vi "Translate Hub Coords.vi"(8 "TOF":dbl, 10 "Input Velocities":T1, 11 "Hub Coords":cluster{"X":dbl, "Y":dbl}) -> (2 "Distance to Hub (ft)":dbl, 3 "Hub Coords Out":cluster{"X":dbl, "Y":dbl})   [LabVIEW 2025]
uses:
  swerve-template/Type Definitions/Data/Robot Velocities.ctl
panel:
  out "Waveform Chart 2":cluster{"Numeric":sgl, "Numeric":sgl}(graph)
  out "Waveform Chart":dbl(graph)
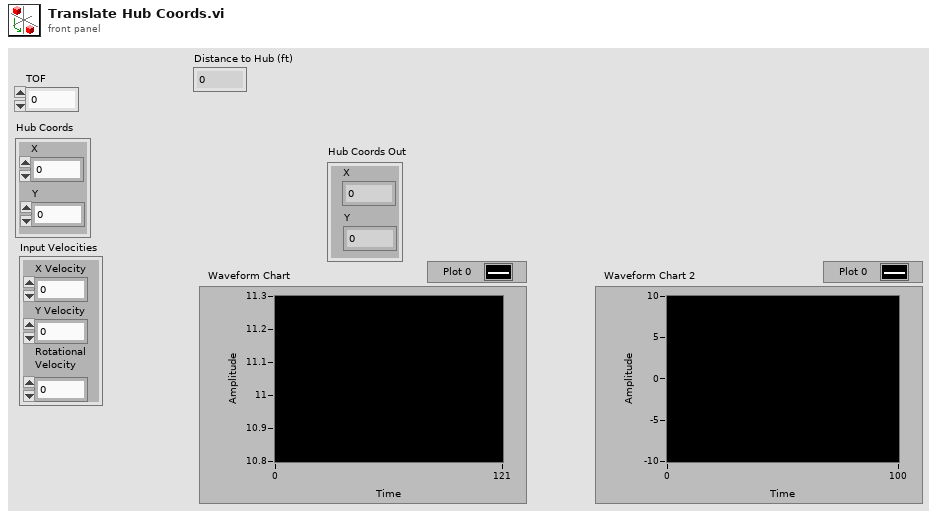
[diagram p1: front panel]
types:
  T1 = typedef "Robot Velocities.ctl" = cluster{"X Velocity":dbl, "Y Velocity":dbl, "Rotational \nVelocity":dbl}
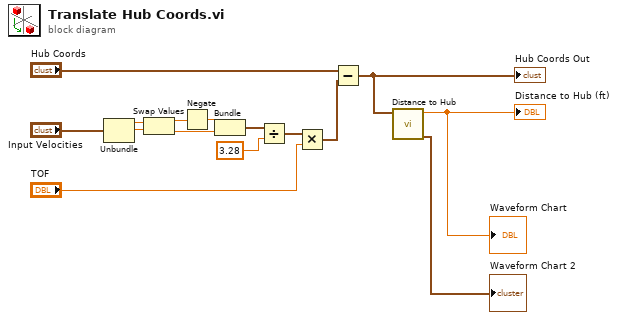
[diagram p0: block diagram]
diagram:
  n1 = Unbundle("Input Velocities") -> ("X Velocity"=w8:dbl, "Y Velocity"=w7:dbl)  [unwired: 1 out]
  n2 = Swap Values(12:w8, 14:w7) -> (1:w4:dbl, 3:w6:dbl)  [unwired: 1 in]
  n3 = Negate(x=w4) -> (-x=w3:dbl)
  n4 = Bundle(w3, w6) -> (w5:cluster{dbl, dbl})  [unwired: 1 in]
  n5 = Divide(x=w5, y=3.28) -> (x/y=w13:cluster{dbl, dbl})
  n6 = Multiply(x=w13, y="TOF") -> (x*y=w9:cluster{dbl, dbl})
  n7 = Subtract(x="Hub Coords", y=w9) -> (x-y=w10:cluster{dbl, dbl})
  "Hub Coords Out" <- w10
  n8 = call "Distance to Hub.vi"("Hub Coords"=w10) -> ("output cluster"=→"Waveform Chart 2":cluster{"Numeric":sgl, "Numeric":sgl}, "Distance to Hub (ft)"=→"Distance to Hub (ft)" →"Waveform Chart":dbl)  [unwired: 8 in, 1 out]
